vi "Relay - Which Chan.vi"() -> (1 "Relay Channel":i32, 2 "Status":string, 3 "Relay":string)   [LabVIEW 2022 SP3]
uses:
  <vilib>/Utility/error.llb/Trim Whitespace One-Sided.vi
  <vilib>/regexp/Match Regular Expression.xnode
panel:
  out "standard output":string
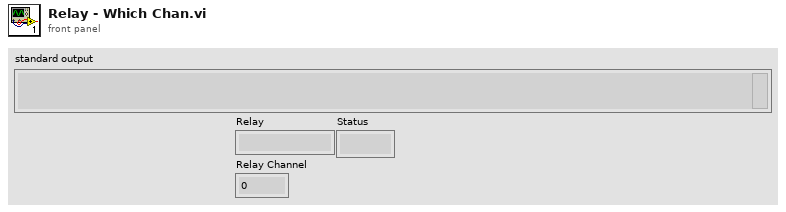
[diagram p1: front panel]
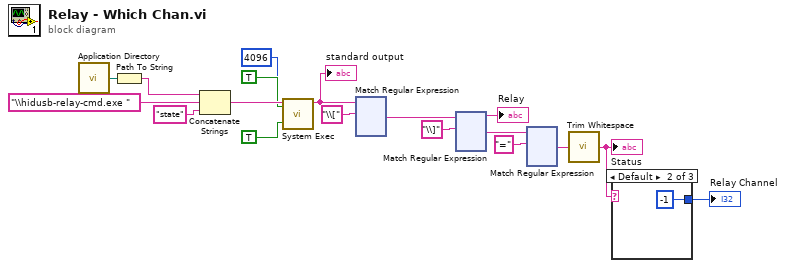
[diagram p0: block diagram]
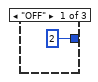
[diagram p2: hidden frame]
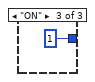
[diagram p3: hidden frame]
diagram:
  n1 = call <vilib>:"Application Directory.vi"() -> ("Application Directory"=w5:path)
  n2 = Path To String(path=w5) -> (string=w4:string)
  n3 = Concatenate Strings(w4, "\\hidusb-relay-cmd.exe " ("command line"), "state") -> (w16:string)
  n4 = call <vilib>:"System Exec.vi"("expected output size  (4096)"=u32 4096, "run minimized? (F)"=TRUE, "wait until completion? (T)"=TRUE, "command line"=w16) -> ("standard output"=w12:string)  [unwired: 4 in, 3 out]
  "standard output" <- w12
  n5 = xnode "Match Regular Expression"("input string"=w12, "regular expression"="\\[") -> ("after match"=w9:string)  [unwired: 4 in, 4 out]
  n6 = xnode "Match Regular Expression"("input string"=w9, "regular expression"="\\]") -> ("before match"=→"Relay":string, "after match"=w6:string)  [unwired: 4 in, 3 out]
  n7 = xnode "Match Regular Expression"("input string"=w6, "regular expression"="=") -> ("after match"=w3:string)  [unwired: 4 in, 4 out]
  n8 = call <vilib>:"Trim Whitespace.vi"("string"=w3) -> ("trimmed string"=w1:string)  [unwired: 1 in]
  "Status" <- w1
  n9 = case shown="Default" w1 {
    tunnel: [2 -1 1] -> w2
    frame "OFF" {
    }
    frame Default {
    }
    frame "ON" {
    }
  }
  "Relay Channel" <- w2
